vi "Next Child Task.vi"(8 "error in (no error)":errorcluster, 10 "Composite Task In":refnum<class "Task Ancestor.lvclass">, 11 "Composite Task Iterator in":refnum<class "Composite Task Iterator.lvclass">) -> (0 "error out":errorcluster, 1 "Child Key":i64=-9000000000000000000 format="%.0p", 2 "Composite Task Out":refnum<class "Task Ancestor.lvclass">, 3 "Composite Task Iterator out":refnum<class "Composite Task Iterator.lvclass">, 4 "Child Task Out":refnum<class "Task Ancestor.lvclass">, 6 "Last":bool)   [LabVIEW 2024, in "Composite Task Iterator.lvclass"]
uses:
  Composite Task Iterator.lvclass
  Ancestor Class/Task/Task Ancestor/Task Ancestor.lvclass
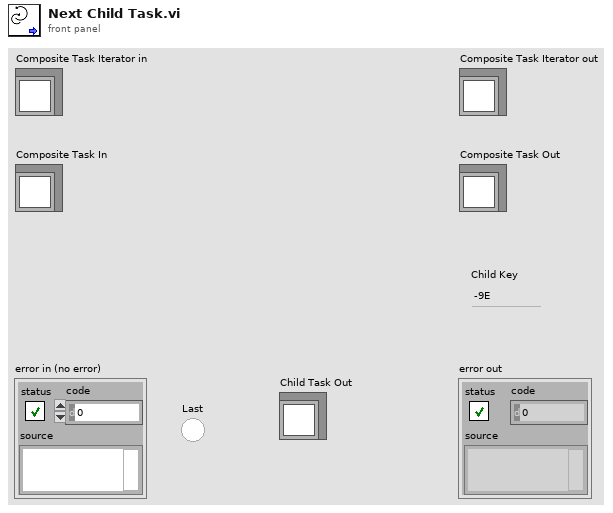
[diagram p1: front panel]
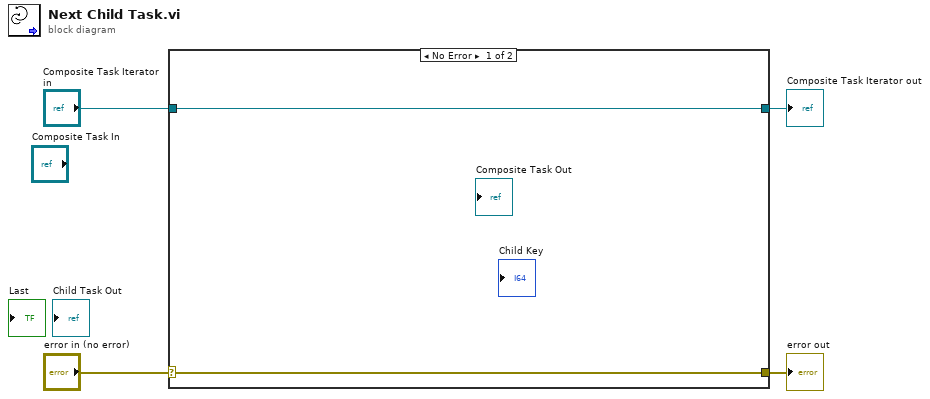
[diagram p0: block diagram]
diagram:
  n1 = case shown="No Error" "error in (no error)" {
    selector: "error in (no error)" -> [w5 w8]
    tunnel: [w5 w8] -> w3
    tunnel: [w6 w7] -> w1
    tunnel: "Composite Task Iterator in" -> [w6 w7]
    frame No Error {
    }
    frame Error {
    }
  }
  "error out" <- w3
  "Composite Task Iterator out" <- w1
